vi "ReadDictionary - private.vi"(8 "error in (no error)":errorcluster, 11 "Dictionary File Path":path) -> (0 "error out":errorcluster, 2 "Dictionary":string[][](array[string]), 3 "Dictionary File Path out":path)   [LabVIEW 2017, in "JKI Simple Localization.lvlib"]
uses:
  API/JKI Simple Localization.lvlib
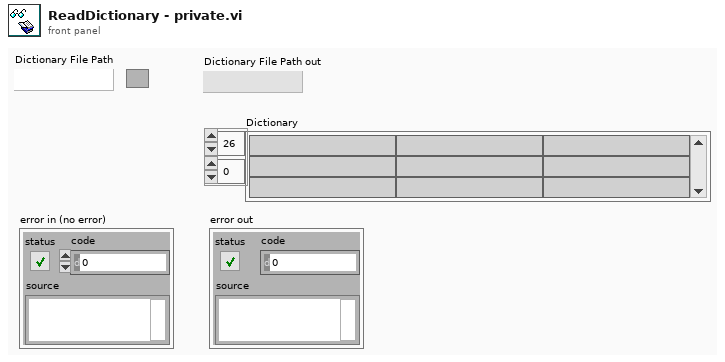
[diagram p1: front panel]
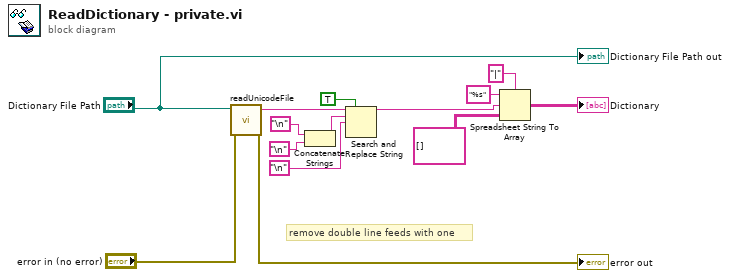
[diagram p0: block diagram]
diagram:
  # "remove double line feeds with one"
  n1 = call "readUnicodeFile.vi"("error in (no error)"="error in (no error)", "File Path"="Dictionary File Path") -> ("error out"=→"error out":errorcluster, "ASCII String"=w5:string)  [unwired: 8 in]
  n2 = Concatenate Strings("\n" ("Line Feed Constant"), "\n" ("Line Feed Constant")) -> (w8:string)
  n3 = Search and Replace String(replace all?=TRUE ("replace all? (F)"), input string=w5, search string=w8, replace string="\n" ("Line Feed Constant")) -> (result string=w4:string)  [unwired: 4 in, 3 out]
  n4 = Spreadsheet String To Array(delimiter (Tab)="|", format string="%s", spreadsheet string=w4, array type (2D Dbl)=string[][] [] ("all rows")) -> (array=→"Dictionary":string[][])
  "Dictionary File Path out" <- "Dictionary File Path"
